vi "Save_TDMS.vi"(8 "error in (no error)":errorcluster, 10 "?":T1={"maximum value"=8.0, "minimum value"=-5.0, "samples per channel"=100.0, "Sample rate"=1000.0, "physical channels"="Dev1/ai0", "sample mode"=10123, "Itterations"=0, "source"="OnboardClock"} {"sample mode" items=["Finite Samples"=10178, "Continuous Samples"=10123, "Hardware Timed Single Point"=12522]; "Sample rate" format="%0.2f"; "minimum value" format="%0.2f"; "maximum value" format="%0.2f"}, 11 "Waveform":waveform(dbl)) -> (0 "error out":errorcluster, 3 "Numeric":u16)   [LabVIEW 2020]
uses:
  DAQmx_settings.ctl
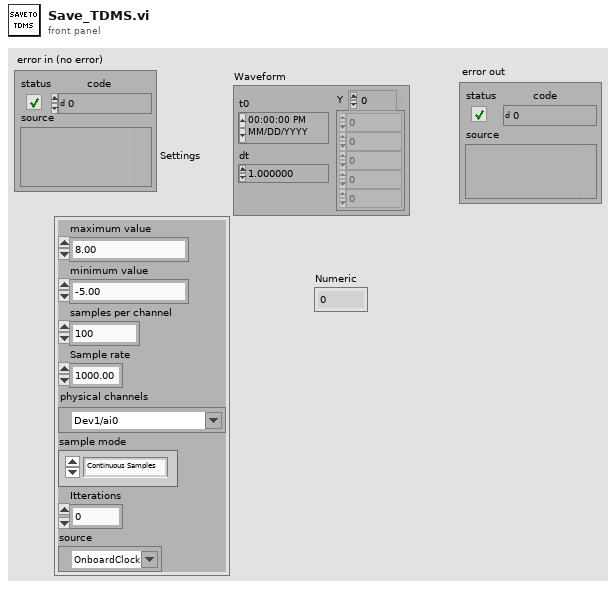
[diagram p1: front panel]
types:
  T1 = typedef "DAQmx_settings.ctl" = cluster{"maximum value":dbl, "minimum value":dbl, "samples per channel":dbl, "Sample rate":dbl, "physical channels":tag, "sample mode":i32, "Itterations":u16, "source":tag}
  T2 = enum16{"open", "open or create", "create or replace", "create", "open (read-only)"}
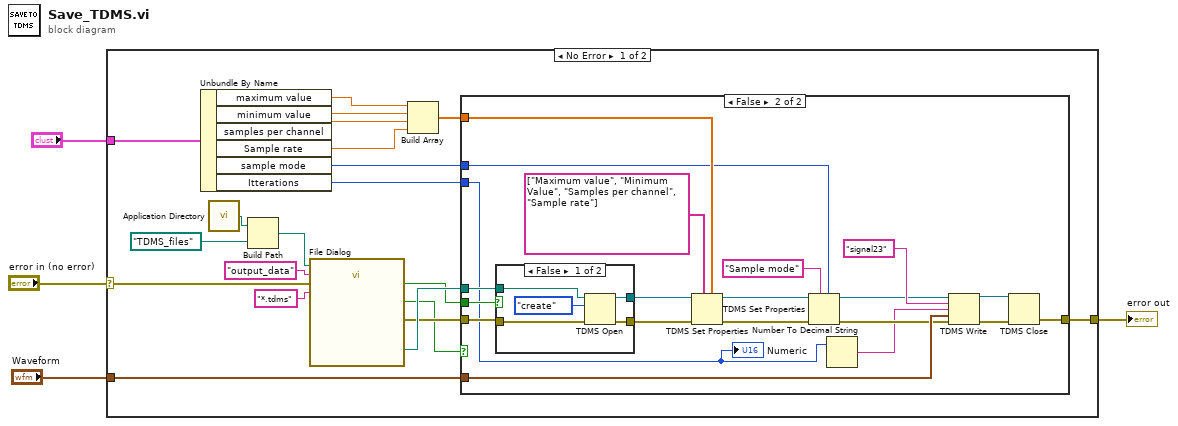
[diagram p0: block diagram]
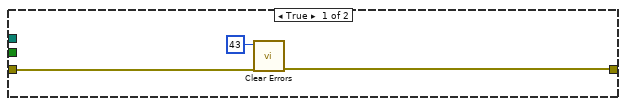
[diagram p2: hidden frame]
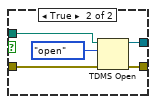
[diagram p3: hidden frame]
diagram:
  n1 = case shown="No Error" "error in (no error)" {
    selector: "error in (no error)" -> [w24 w58]
    tunnel: [w13 w58] -> w3
    tunnel: "Waveform" -> [w11 _]
    tunnel: "?" -> [w18 _]
    frame No Error {
      n2 = Unbundle By Name(w18) -> ("maximum value"=w17:dbl, "minimum value"=w16:dbl, "samples per channel"=w15:dbl, "Sample rate"=w14:dbl, "sample mode"=w6:i32, "Itterations"=w5:u16)
      n3 = call <vilib>:"Application Directory.vi"() -> ("Application Directory"=w23:path)
      n4 = Build Path(base path=w23, name or relative path=path "TDMS_files") -> (appended path=w22:path)
      n5 = call "File Dialog"("start path"=w22, "default name"="output_data", "error in"=w24, "pattern (all files)"="*.tdms") -> ("selected path"=w10:path, "exists"=w8:bool, "cancelled"=w7:bool, "error out"=w9:errorcluster)  [unwired: 8 in]
      n6 = Build Array(w17, w16, w15, w14) -> (w12:dbl[])
      n7 = case shown="False" w7 {
        tunnel: [w25 w40] -> w13
        tunnel: w12 -> [_ w39]
        tunnel: w11 -> [_ w38]
        tunnel: w10 -> [_ w37]
        tunnel: w9 -> [w26 w36]
        tunnel: w8 -> [_ w35]
        tunnel: w6 -> [_ w33]
        tunnel: w5 -> [_ w28]
        frame True {
          n8 = call <vilib>:"Clear Errors.vi"("error in (no error)"=w26, "specific error code to clear (0: all)"=43) -> ("error out"=w25:errorcluster)  [unwired: 4 in, 1 out]
        }
        frame False {
          n9 = case shown="False" w35 {
            tunnel: w36 -> [w51 w57]
            tunnel: [w50 w56] -> w43
            tunnel: w37 -> [w48 w55]
            tunnel: [w49 w53] -> w44
            frame False {
              n10 = TDMS Open(8:w51, 10:T2."create" ("operation (0:open)"), 11:w48) -> (0:w50:errorcluster, 3:w49:refnum<k34>)  [unwired: 4 in]
            }
            frame True {
              n11 = TDMS Open(8:w57, 10:T2."open" ("operation (0:open)"), 11:w55) -> (0:w56:errorcluster, 3:w53:refnum<k34>)  [unwired: 4 in]
            }
          }
          n12 = TDMS Set Properties(5:w39, 7:string[] ["Maximum value", "Minimum Value", "Samples per channel", "Sample rate"] ("property names"), 8:w43, 11:w44) -> (0:w45:errorcluster, 3:w34:refnum<k34>)  [unwired: 2 in, 2 out]
          n13 = TDMS Set Properties(5:w33, 7:"Sample mode", 8:w45, 11:w34) -> (0:w30:errorcluster, 3:w31:refnum<k34>)  [unwired: 2 in, 2 out]
          n14 = Number To Decimal String(number=w28) -> (decimal integer string=w29:string)  [unwired: 1 in]
          n15 = TDMS Write(0:w31, 5:"signal23" ("group name in (Untitled)"), 7:w29, 9:w38, 11:w30) -> (4:w46:refnum<k34>, 15:w47:errorcluster)  [unwired: 1 in, 2 out]
          n16 = TDMS Close(8:w47, 11:w46) -> (0:w40:errorcluster)  [unwired: 1 out]
          "Numeric" <- w28
        }
      }
    }
    frame Error {
    }
  }
  "error out" <- w3
